vi "Transmit.vi"(8 "error in (no error)":errorcluster, 10 "Transfer Group in":refnum<class "Transfer Group.lvclass">, 11 "UDPlog Transceiver in":refnum<class "UDPlog Transceiver.lvclass">) -> (0 "error out":errorcluster, 2 "Transfer Group out":refnum<class "Transfer Group.lvclass">, 3 "UDPlog Transceiver out":refnum<class "UDPlog Transceiver.lvclass">)   [LabVIEW 2023, in "UDPlog.lvlib" / "UDPlog Transceiver.lvclass"]
uses:
  UDPlog Transceiver.lvclass
  UDPlog Transceiver.lvclass/UDPlog Transceiver.ctl
  <vilib>/AddOns/VeriStand Custom Device Scripting APIs/Data Sharing Framework/DSF Core.lvlibp/Classes/Transfer Group/Transfer Group.lvclass
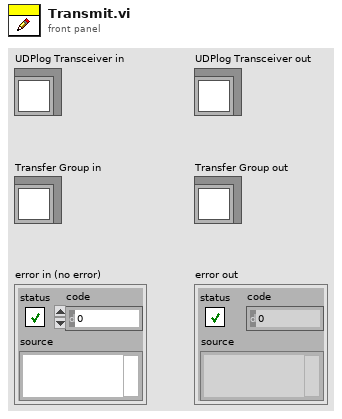
[diagram p1: front panel]
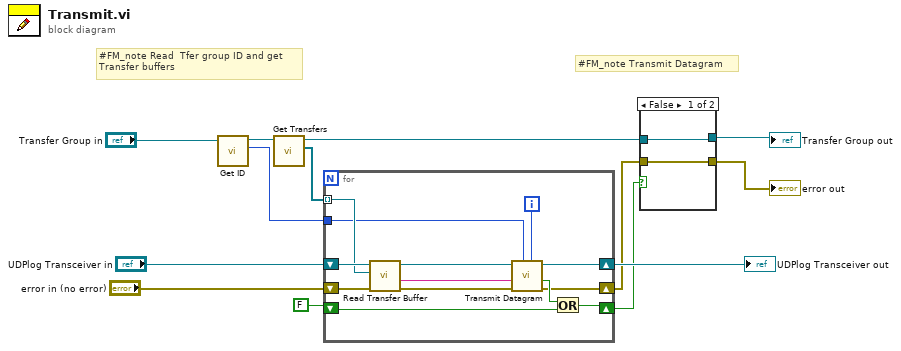
[diagram p0: block diagram]
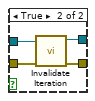
[diagram p2: hidden frame]
diagram:
  # "#FM_note Transmit Datagram"
  # "#FM_note Read  Tfer group ID and get\nTransfer buffers"
  n1 = call <vilib>:"Get ID.vi"("Transfer Group in"="Transfer Group in") -> ("id"=w7:i32, "Transfer Group out"=w12:refnum<class "Transfer Group.lvclass">)  [unwired: 9 in]
  n2 = call <vilib>:"Get Transfers.vi"("Transfer Group in"=w12) -> ("Transfers"=w8:refnum<class "Transfer.lvclass">[], "Transfer Group out"=w11:refnum<class "Transfer Group.lvclass">)  [unwired: 9 in]
  n3 = for {
    tunnel: w8 -> [w24] mode=indexing
    tunnel: w7 -> [w15]
    shift-right: [w18] -> w4
    shift-left: "UDPlog Transceiver in" -> [w26]
    shift-right: [w19] -> w3
    shift-left: "error in (no error)" -> [w25]
    shift-right: [w21] -> w1
    shift-left: FALSE -> [w22]
    i -> [w14]
    n4 = call "Read Transfer Buffer.vi"("error in (no error)"=w25, "Transfer"=w24, "UDPlog Transceiver in"=w26) -> ("error out"=w20:errorcluster, "data"=w16:string, "UDPlog Transceiver out"=w17:refnum<class "UDPlog Transceiver.lvclass">)  [unwired: 6 in]
    n5 = call "Transmit Datagram.vi"("transfer id"=w14, "transfer group id"=w15, "error in (no error)"=w20, "transfer data"=w16, "UDPlog Transceiver in"=w17) -> ("error out"=w19:errorcluster, "timed out?"=w23:bool, "UDPlog Transceiver out"=w18:refnum<class "UDPlog Transceiver.lvclass">)  [unwired: 4 in]
    n6 = Or(x=w23, y=w22) -> (x .or. y?=w21:bool)
  }
  "UDPlog Transceiver out" <- w4
  n7 = case shown="False" w1 {
    tunnel: w11 -> [w28 w32]
    tunnel: [w28 w31] -> w10
    tunnel: [w27 w30] -> w9
    tunnel: w3 -> [w27 w29]
    frame False {
    }
    frame True {
      n8 = call <vilib>:"Invalidate Iteration.vi"("error in (no error)"=w29, "Transfer Group in"=w32) -> ("error out"=w30:errorcluster, "Transfer Group out"=w31:refnum<class "Transfer Group.lvclass">)  [unwired: 8 in]
    }
  }
  "error out" <- w9
  "Transfer Group out" <- w10
